vi "FPGAThrust.vi"() -> (4 "Mod1-9237/AI0":sgl, 6 "Mod1-9237/AI1":sgl, 8 "Load 1: Force (lbf)":sgl, 10 "Load 2: Force (lbf)":sgl, 15 "Total Thrust Force (lbf)":sgl)   [LabVIEW 2019]
uses:
  <vilib>/rvi/eio/common/nirviEmuTemplateMethod_errors.vi
  <vilib>/eio/EIONode/EIONode.xnode
  <vilib>/rvi/Analysis/measure/butterworth/XNode/niFpgaButterworthFilter.xnode
panel:
  # "READ Thrust Sensors"
  # "Futek LCM375 10klbf Tension"
  # "(Volts)"
  # "Load 1: S/N 702360"
  # "(Volts)"
  # "Load 2: S/N 702359"
  # "S/N 702360 Calibration Data"
  # "S/N 702359 Calibration Data"
  # "L1 Excitation = 9.99 Vdc"
  # "L2 Excitation = 9.99 Vdc"
  # "L1 Calib Pt -1 (<0) = 2.1364e-4 lbf/(mV/V)"
  # "L2 Calib Pt -1 (<0) = 2.1316e-4 lbf/(mV/V)"
  # "L1 Calib Pt 0 (0-2k) = 2.1515e-4 lbf/(mV/V)"
  # "L2 Calib Pt 0 (0-2k) = 2.1370e-4 lbf/(mV/V)"
  # "L1 Calib Pt 1 (2k-4k) = 2.1560e-4 lbf/(mV/V)"
  # "L2 Calib Pt 1 (2k-4k) = 2.1445e-4 lbf/(mV/V)"
  # "L1 Calib Pt 2 (4k-6k) = 2.1585e-4 lbf/(mV/V)"
  # "L2 Calib Pt 2 (4k-6k) = 2.1505e-4 lbf/(mV/V)"
  # "L1 Calib Pt 3 (6k-8k) = 2.1685e-4 lbf/(mV/V)"
  # "L2 Calib Pt 3 (6k-8k) = 2.1525e-4 lbf/(mV/V)"
  # "L1 Calib Pt 4 (8k-10k) = 2.1566e-4 lbf/(mV/V)"
  # "L2 Calib Pt 4 (8k-10k) = 2.1620e-4 lbf/(mV/V)"
  # "L1 Factory Zero = 0.0044 mV/V"
  # "L2 Factory Zero = 0.0043 mV/V"
  # "L1 Nominal Zero = 0.00667 mV/V"
  # "L2 Nominal Zero = 0.00572 mV/V"
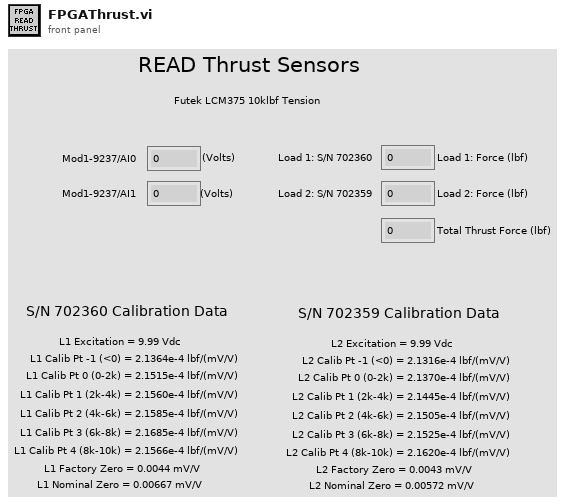
[diagram p1: front panel]
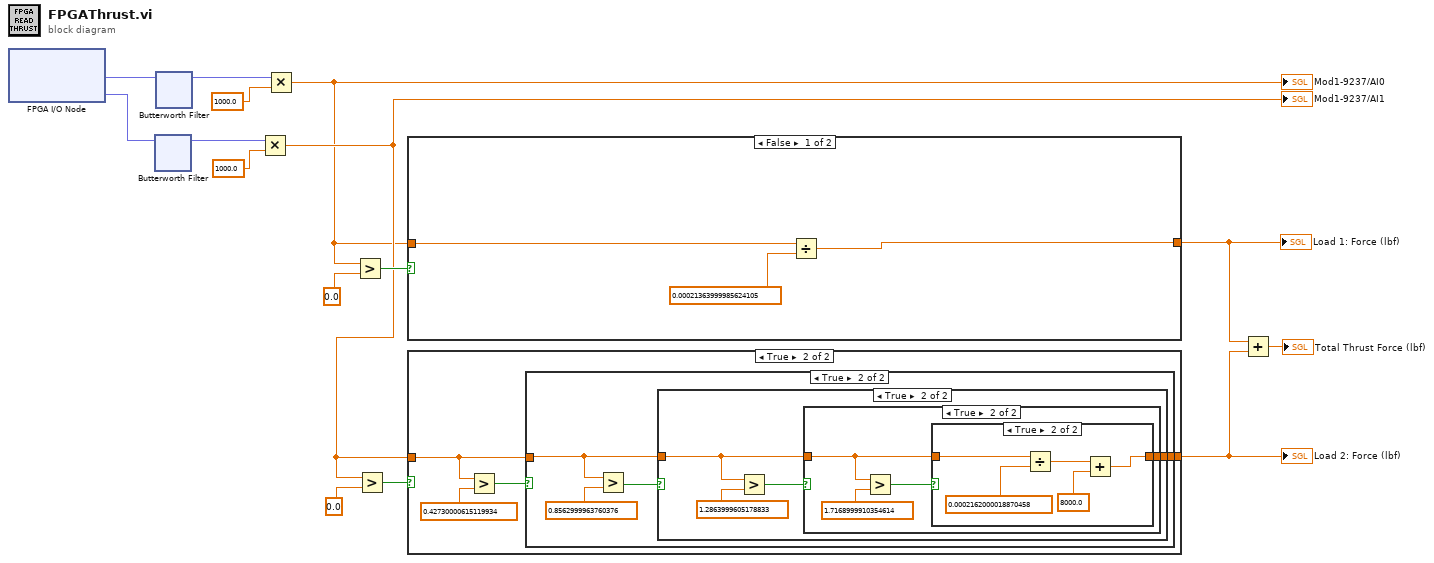
[diagram p0: block diagram]
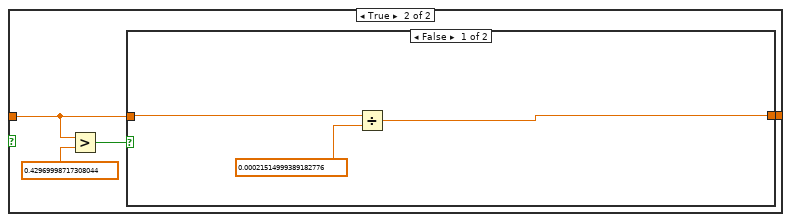
[diagram p2: hidden frame]
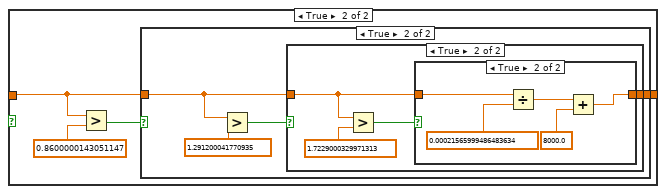
[diagram p3: hidden frame]
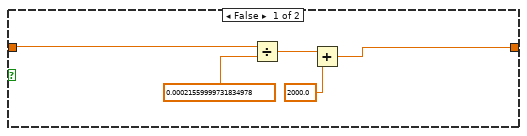
[diagram p4: hidden frame]
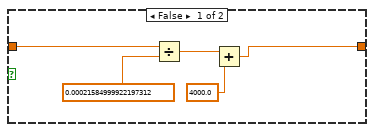
[diagram p5: hidden frame]
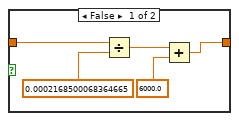
[diagram p6: hidden frame]
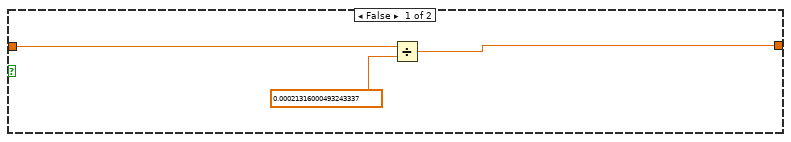
[diagram p7: hidden frame]
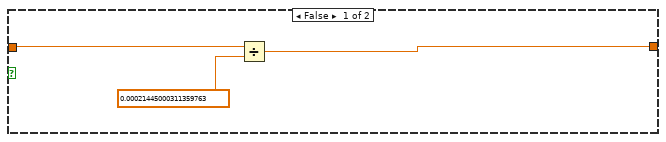
[diagram p8: hidden frame]
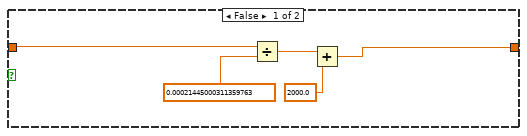
[diagram p9: hidden frame]
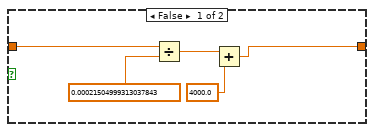
[diagram p10: hidden frame]
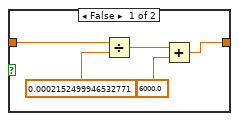
[diagram p11: hidden frame]
diagram:
  n1 = xnode "FPGA I/O Node"() -> ("Mod1/AI0"=w5:fxp<+/-,24,-4>, "Mod1/AI1"=w3:fxp<+/-,24,-4>)  [unwired: 2 in, 2 out]
  n2 = xnode "Butterworth Filter"("input data"=w3) -> ("output data"=w4:fxp<+/-,28,0>)  [unwired: 2 in]
  n3 = xnode ("Butterworth Filter")("input data"=w5) -> ("output data"=w6:fxp<+/-,28,0>)  [unwired: 2 in]
  n4 = Multiply(x=w4, y=sgl 1000.0) -> (x*y=w8:sgl)
  "Mod1-9237/AI1" <- w8
  n5 = Multiply(x=w6, y=sgl 1000.0) -> (x*y=w7:sgl)
  "Mod1-9237/AI0" <- w7
  n6 = Greater?(x=w7, y=sgl 0.0) -> (0:w13:bool)
  n7 = Greater?(x=w8, y=sgl 0.0) -> (0:w14:bool)
  n8 = case shown="False" w13 {
    tunnel: w7 -> [w17 w22]
    tunnel: [w16 w19] -> w1
    frame False {
      n9 = Divide(x=w17, y=sgl 0.00021364) -> (x/y=w16:sgl)
    }
    frame True {
      n10 = Greater?(x=w22, y=sgl 0.4297) -> (0:w21:bool)
      n11 = case shown="False" w21 {
        tunnel: w22 -> [w24 w27]
        tunnel: [w23 w26] -> w19
        frame False {
          n12 = Divide(x=w24, y=sgl 0.00021515) -> (x/y=w23:sgl)
        }
        frame True {
          n13 = Greater?(x=w27, y=sgl 0.86) -> (0:w28:bool)
          n14 = case shown="True" w28 {
            tunnel: w27 -> [w30 w35]
            tunnel: [w32 w36] -> w26
            frame False {
              n15 = Divide(x=w30, y=sgl 0.0002156) -> (x/y=w34:sgl)
              n16 = Add(x=w34, y=sgl 2000.0) -> (x+y=w32:sgl)
            }
            frame True {
              n17 = Greater?(x=w35, y=sgl 1.2912) -> (0:w37:bool)
              n18 = case shown="True" w37 {
                tunnel: w35 -> [w40 w44]
                tunnel: [w39 w45] -> w36
                frame False {
                  n19 = Divide(x=w40, y=sgl 0.00021585) -> (x/y=w43:sgl)
                  n20 = Add(x=w43, y=sgl 4000.0) -> (x+y=w39:sgl)
                }
                frame True {
                  n21 = Greater?(x=w44, y=sgl 1.7229) -> (0:w46:bool)
                  n22 = case shown="True" w46 {
                    tunnel: w44 -> [w49 w57]
                    tunnel: [w48 w53] -> w45
                    frame False {
                      n23 = Divide(x=w49, y=sgl 0.00021685) -> (x/y=w52:sgl)
                      n24 = Add(x=w52, y=sgl 6000.0) -> (x+y=w48:sgl)
                    }
                    frame True {
                      n25 = Divide(x=w57, y=sgl 0.00021566) -> (x/y=w55:sgl)
                      n26 = Add(x=w55, y=sgl 8000.0) -> (x+y=w53:sgl)
                    }
                  }
                }
              }
            }
          }
        }
      }
    }
  }
  "Load 1: Force (lbf)" <- w1
  n27 = case shown="True" w14 {
    tunnel: w8 -> [w59 w64]
    tunnel: [w58 w61] -> w2
    frame False {
      n28 = Divide(x=w59, y=sgl 0.00021316) -> (x/y=w58:sgl)
    }
    frame True {
      n29 = Greater?(x=w64, y=sgl 0.4273) -> (0:w63:bool)
      n30 = case shown="True" w63 {
        tunnel: w64 -> [w66 w69]
        tunnel: [w65 w68] -> w61
        frame False {
          n31 = Divide(x=w66, y=sgl 0.00021445) -> (x/y=w65:sgl)
        }
        frame True {
          n32 = Greater?(x=w69, y=sgl 0.8563) -> (0:w70:bool)
          n33 = case shown="True" w70 {
            tunnel: w69 -> [w72 w77]
            tunnel: [w74 w78] -> w68
            frame False {
              n34 = Divide(x=w72, y=sgl 0.00021445) -> (x/y=w76:sgl)
              n35 = Add(x=w76, y=sgl 2000.0) -> (x+y=w74:sgl)
            }
            frame True {
              n36 = Greater?(x=w77, y=sgl 1.2864) -> (0:w79:bool)
              n37 = case shown="True" w79 {
                tunnel: w77 -> [w82 w86]
                tunnel: [w81 w87] -> w78
                frame False {
                  n38 = Divide(x=w82, y=sgl 0.00021505) -> (x/y=w85:sgl)
                  n39 = Add(x=w85, y=sgl 4000.0) -> (x+y=w81:sgl)
                }
                frame True {
                  n40 = Greater?(x=w86, y=sgl 1.7169) -> (0:w88:bool)
                  n41 = case shown="True" w88 {
                    tunnel: w86 -> [w91 w99]
                    tunnel: [w90 w95] -> w87
                    frame False {
                      n42 = Divide(x=w91, y=sgl 0.00021525) -> (x/y=w94:sgl)
                      n43 = Add(x=w94, y=sgl 6000.0) -> (x+y=w90:sgl)
                    }
                    frame True {
                      n44 = Divide(x=w99, y=sgl 0.0002162) -> (x/y=w97:sgl)
                      n45 = Add(x=w97, y=sgl 8000.0) -> (x+y=w95:sgl)
                    }
                  }
                }
              }
            }
          }
        }
      }
    }
  }
  "Load 2: Force (lbf)" <- w2
  n46 = Add(x=w1, y=w2) -> (x+y=→"Total Thrust Force (lbf)":sgl)
